vi "D-триггер.vi"(2 "C":bool, 3 "D":bool) -> (0 "not Q":bool, 1 "Q":bool)   [LabVIEW 2012]
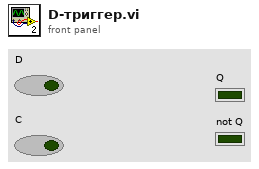
[diagram p1: front panel]
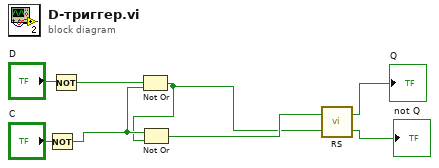
[diagram p0: block diagram]
diagram:
  n1 = Not(x="C") -> (.not. x?=w7:bool)
  n2 = Not(x="D") -> (.not. x?=w5:bool)
  n3 = Not Or(1:w7, 2:w5) -> (0:w3:bool)
  n4 = Not Or(1:w3, 2:w7) -> (0:w4:bool)
  n5 = call "RS.vi"("S"=w3, "R"=w4) -> ("not Q"=→"not Q":bool, "Q"=→"Q":bool)
